vi "3-8.vi"(9 "Min Temp":dbl, 10 "Max Temp":dbl, 11 "Current Temp":dbl) -> (1 "Warning?":bool, 2 "Warning Text":string)   [LabVIEW 2014]
doc: "This VI is an exercise in the LabVIEW Core I course. In this exercise, you generate appropriate strings for Freeze, Heat Stroke, and High Wind warnings, and combinations of the warnings."
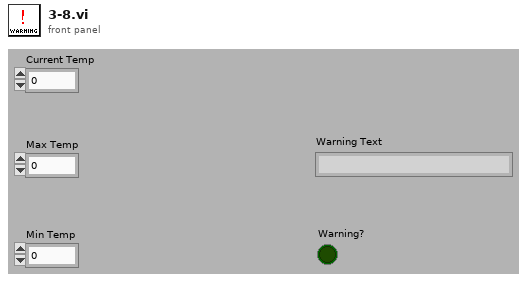
[diagram p1: front panel]
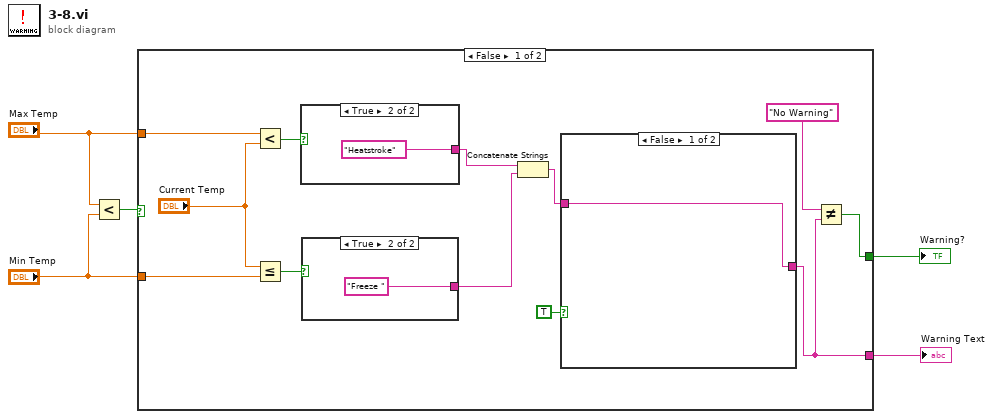
[diagram p0: block diagram]
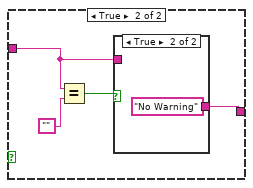
[diagram p2: hidden frame]
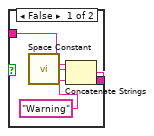
[diagram p3: hidden frame]
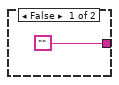
[diagram p4: hidden frame]
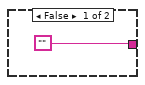
[diagram p5: hidden frame]
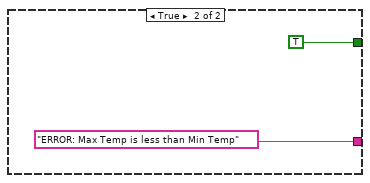
[diagram p6: hidden frame]
diagram:
  n1 = Less?(x="Max Temp", y="Min Temp") -> (x < y?=w1:bool)
  n2 = case shown="False" w1 {
    tunnel: [w8 TRUE] -> w5
    tunnel: [w7 "ERROR: Max Temp is less than Min Temp"] -> w4
    tunnel: "Max Temp" -> [w14 _]
    tunnel: "Min Temp" -> [w13 _]
    frame False {
      n3 = Less?(x=w14, y="Current Temp") -> (x < y?=w15:bool)
      n4 = Less Or Equal?(x="Current Temp", y=w13) -> (x <= y?=w17:bool)
      n5 = case shown="True" w15 {
        tunnel: ["" "Heatstroke"] -> w12
        frame False {
        }
        frame True {
        }
      }
      n6 = case shown="True" w17 {
        tunnel: ["" "Freeze "] -> w11
        frame False {
        }
        frame True {
        }
      }
      n7 = Concatenate Strings(w12, w11) -> (w10:string)
      n8 = case shown="False" TRUE {
        tunnel: w10 -> [w18 w20]
        tunnel: [w18 w19] -> w7
        frame False {
        }
        frame True {
          n9 = Equal?(x=w20, y="") -> (x = y?=w21:bool)
          n10 = case shown="True" w21 {
            tunnel: w20 -> [w23 _]
            tunnel: [w26 "No Warning"] -> w19
            frame False {
              n11 = call <vilib>:"Space Constant.vi"() -> ("String"=w24:string)
              n12 = Concatenate Strings(w23, w24, "Warning") -> (w26:string)
            }
            frame True {
            }
          }
        }
      }
      n13 = Not Equal?(x="No Warning", y=w7) -> (x != y?=w8:bool)
    }
    frame True {
    }
  }
  "Warning Text" <- w4
  "Warning?" <- w5
